vi "basic_arduino_comm.vi"() -> ()   [LabVIEW 2022 SP3]
doc: "This example performs writes and reads on a serial port, as directed by the user. You can press the Write and Read buttons, and change the Read Count, while the example is running.\n\nThe parameters set for the serial port must match the parameters of the connected instrument or device. In this example, the Read Count parameter specifies the number of bytes that the serial port reads. If there were more bytes at the port than the specified number, those bytes would not be read. If there were less bytes at the port than the specified number, you would receive a timeout error.\n\nThis example expands upon the flow control options for XON and XOFF, allowing the user to choose those control characters. Also, the user can enable or disable a termination character. Some devices require a termination character in order to identify the end of command strings. Some devices send a termination character to signify the end of data to be read. This example shows how you can end the Read operation once a termination character is detected in the buffer and/or append a termination character at the end of the Write data."
uses:
  <vilib>/Instr/_visa.llb/VISA Configure Serial Port (Instr).vi
panel:
  in  "Enable Termination\nChar (T)":bool=TRUE
  in  "termination char\n(0xA = '\\n' = LF)":u8=10 format="%.0x"
  out "Waveform Chart":i32(graph)
  in  "Stop":bool
  in  "Read Count":u32=1000
  in  "Start Reading":bool
  in  "VISA resource name":refnum<visa-resource-name>="COM1"
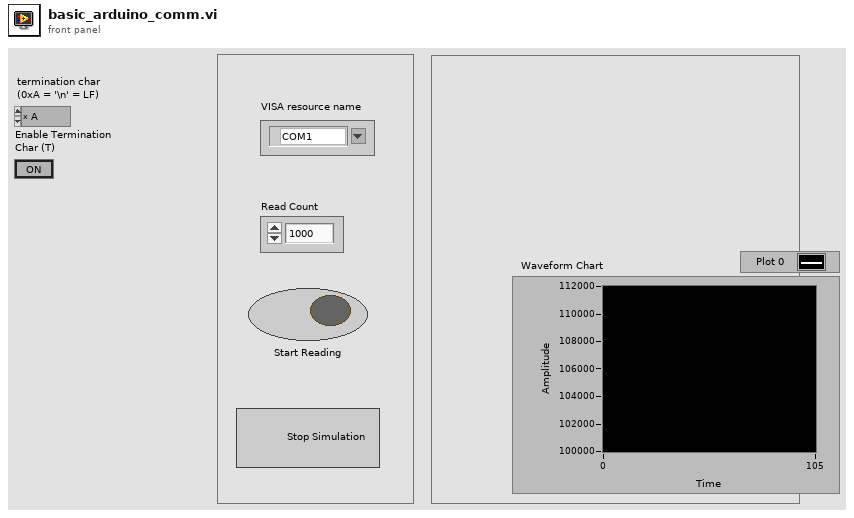
[diagram p1: front panel]
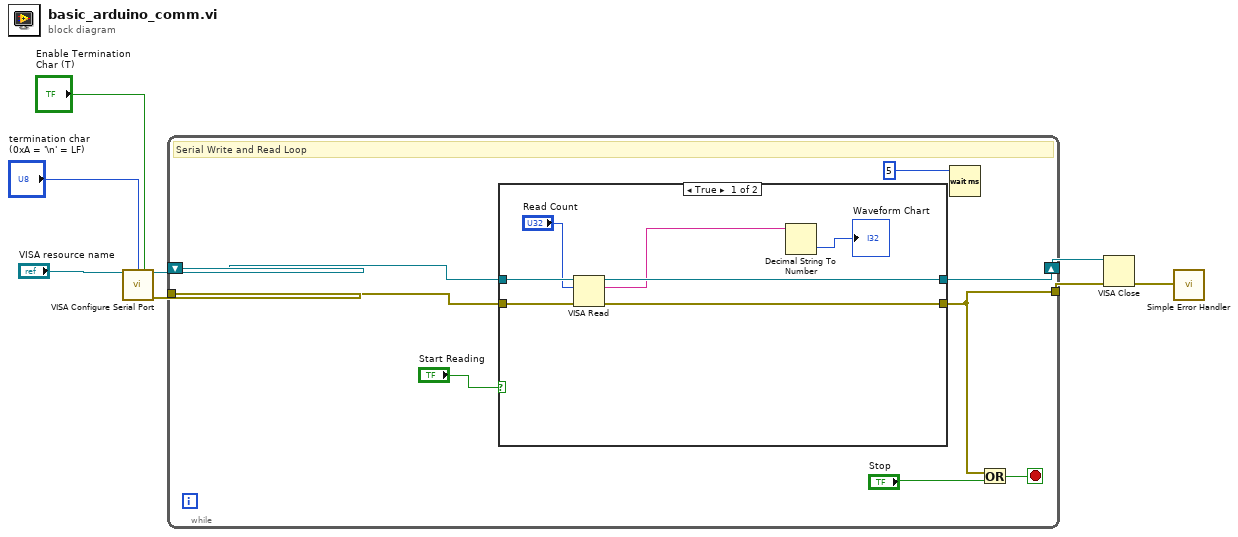
[diagram p0: block diagram]
diagram:
  n1 = call-poly "VISA Configure Serial Port"("VISA resource name"="VISA resource name", "termination char\n(0xA = '\\n' = LF)"="termination char\n(0xA = '\\n' = LF)", "Enable Termination\nChar (T)"="Enable Termination\nChar (T)") -> ("VISA resource name out"=w4:refnum<visa-resource-name>, "error out"=w3:errorcluster)  [unwired: 7 in, 4 out]
  n2 = while {
    shift-right: [w16] -> w5
    shift-left: w4 -> [w13]
    tunnel: w3 -> [w12]
    tunnel: [w14] -> w6
    stop <- w9 stop-if-true
    # "Serial Write and Read Loop"
    n3 = case shown="True" "Start Reading" {
      tunnel: [w21 w25] -> w16
      tunnel: w13 -> [w23 w25]
      tunnel: [w19 w24] -> w14
      tunnel: w12 -> [w22 w24]
      frame True {
        n4 = VISA Read(VISA resource name=w23, byte count="Read Count", error in (no error)=w22) -> (VISA resource name out=w21:refnum<visa-resource-name>, read buffer=w17:string, error out=w19:errorcluster)  [unwired: 1 out]
        n5 = Decimal String To Number(string=w17) -> (number=→"Waveform Chart":i32)  [unwired: 2 in, 1 out]
      }
      frame False {
      }
    }
    n6 = Wait (ms)(milliseconds to wait=u32 5) -> ()  [unwired: 1 out]
    n7 = Or(x=w14, y="Stop") -> (x .or. y?=w9:bool)
  }
  n8 = VISA Close(VISA resource name=w5, error in (no error)=w6) -> (error out=w7:errorcluster)
  n9 = call <vilib>:"Simple Error Handler.vi"("error in (no error)"=w7) -> ()  [unwired: 1 in, 8 out]
